vi "LV_sender.vi"() -> ()   [LabVIEW 2019]
panel:
  in  "stop":bool
  in  "vooruit":bool
  in  "achteruit":bool
  in  "links":bool
  in  "rechts":bool
  in  "linksvooruit":bool
  in  "rechtsvooruit":bool
  in  "rechtsachter":bool
  in  "linksachter":bool
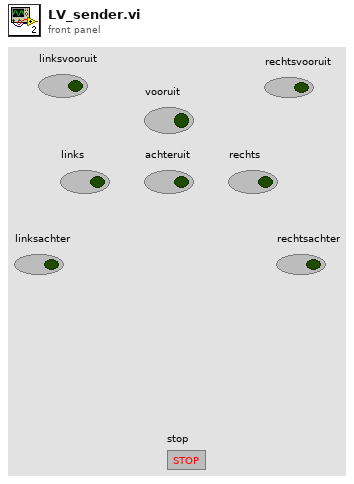
[diagram p1: front panel]
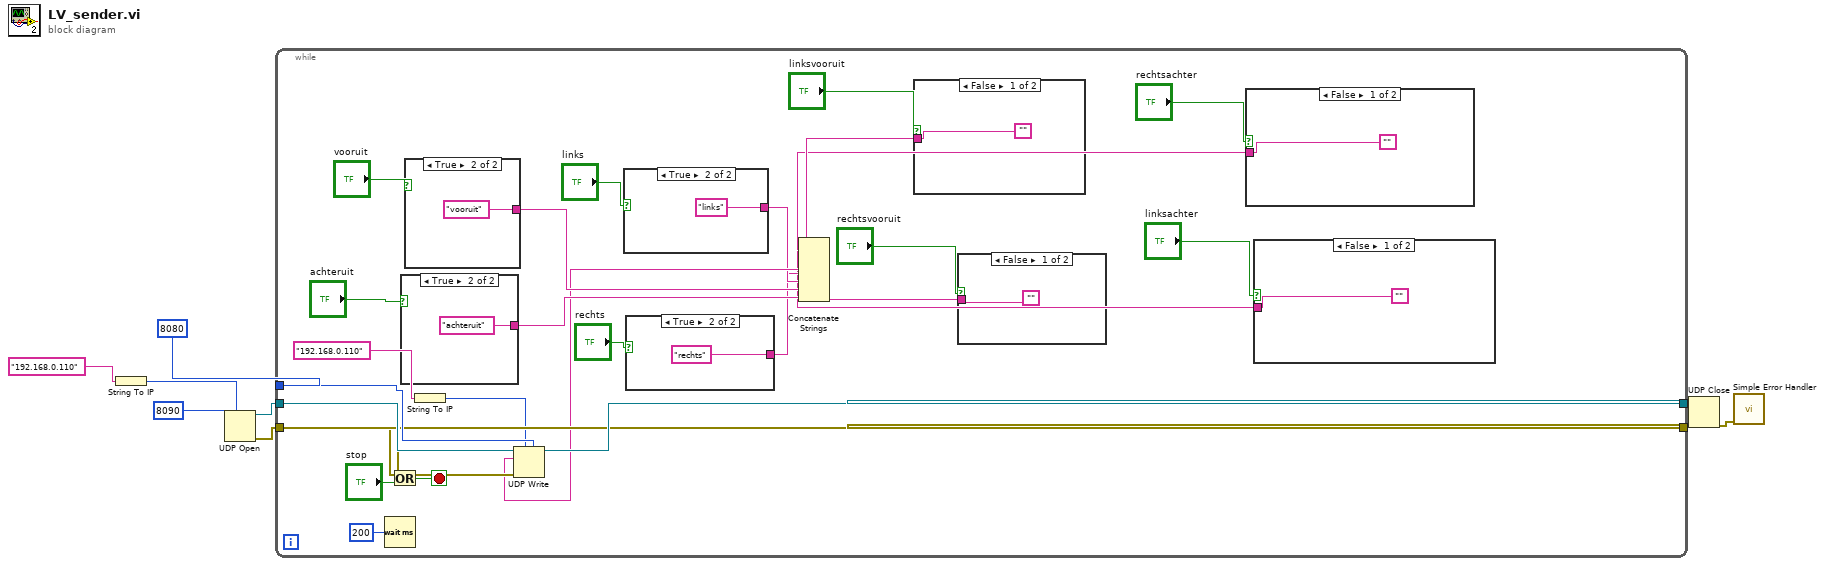
[diagram p0: block diagram]
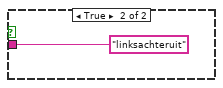
[diagram p2: hidden frame]
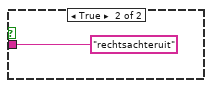
[diagram p3: hidden frame]
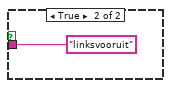
[diagram p4: hidden frame]
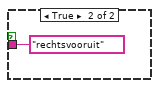
[diagram p5: hidden frame]
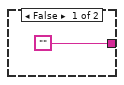
[diagram p6: hidden frame]
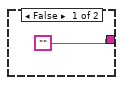
[diagram p7: hidden frame]
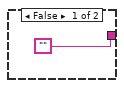
[diagram p8: hidden frame]
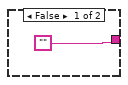
[diagram p9: hidden frame]
diagram:
  n1 = String To IP(1:"192.168.0.110") -> (0:w1:u32)
  n2 = UDP Open(7:w1, 11:8090) -> (port=w8:refnum<k16>, 0:w7:errorcluster)  [unwired: 3 in, 1 out]
  n3 = while {
    tunnel: w8 -> [w36]
    tunnel: w7 -> [w35]
    tunnel: 8080 -> [w31]
    tunnel: [w30] -> w5
    tunnel: [w29] -> w4
    stop <- w33 stop-if-true
    n4 = Wait (ms)(milliseconds to wait=200) -> ()  [unwired: 1 out]
    n5 = case shown="True" "achteruit" {
      tunnel: ["" "achteruit"] -> w25
      frame False {
      }
      frame True {
      }
    }
    n6 = case shown="True" "vooruit" {
      tunnel: ["" "vooruit"] -> w26
      frame False {
      }
      frame True {
      }
    }
    n7 = String To IP(1:"192.168.0.110") -> (0:w22:u32)
    n8 = case shown="True" "links" {
      tunnel: ["" "links"] -> w21
      frame False {
      }
      frame True {
      }
    }
    n9 = case shown="True" "rechts" {
      tunnel: ["" "rechts"] -> w19
      frame False {
      }
      frame True {
      }
    }
    n10 = case shown="False" "linksvooruit" {
      tunnel: ["" "linksvooruit"] -> w15
      frame False {
      }
      frame True {
      }
    }
    n11 = case shown="False" "rechtsvooruit" {
      tunnel: ["" "rechtsvooruit"] -> w16
      frame False {
      }
      frame True {
      }
    }
    n12 = case shown="False" "rechtsachter" {
      tunnel: ["" "rechtsachteruit"] -> w13
      frame False {
      }
      frame True {
      }
    }
    n13 = case shown="False" "linksachter" {
      tunnel: ["" "linksachteruit"] -> w12
      frame False {
      }
      frame True {
      }
    }
    n14 = Concatenate Strings(w12, w13, w15, w16, w19, w21, w26, w25) -> (w24:string)
    n15 = UDP Write(address=w22, port or service name=w31, connection ID=w36, data in=w24, 8:w35) -> (error out=w29:errorcluster, 3:w30:refnum<k16>)  [unwired: 1 in]
    n16 = Or(x=w29, y="stop") -> (x .or. y?=w33:bool)
  }
  n17 = UDP Close(connection ID=w5, 8:w4) -> (error out=w3:errorcluster)  [unwired: 1 out]
  n18 = call <vilib>:"Simple Error Handler.vi"("error in (no error)"=w3) -> ()  [unwired: 4 in, 5 out]
